vi "Open.vi"(8 "error in":errorcluster, 9 "parameters":variant, 10 "file path":path, 11 "CEF_Hierachy Repository in":refnum<class "CEF_HierarchyRepo.lvclass">) -> (0 "error out":errorcluster, 2 "invalid?":bool, 3 "CEF_Hierachy repository out":refnum<class "CEF_HierarchyRepo.lvclass">)   [LabVIEW 2023, in "CEF.lvlib" / "CEF_HierarchyRepo.lvclass"]
doc: "Loads the saved information of the repo. It could load multiple files at the same time. An option to add file versioning could be included in the files, and the code to manage changes would be in this VI.Copyright 2017 National Instruments Corporation\n\nLicensed under the Apache License, Version 2.0 (the \"License\"); you may not use this file except in compliance with the License. You may obtain a copy of the License at http://www.apache.org/licenses/LICENSE-2.0\nUnless required by applicable law or agreed to in writing, software distributed under the License is distributed on an \"AS IS\" BASIS, WITHOUT WARRANTIES OR CONDITIONS OF ANY KIND, either express or implied. See the License for the specific language governing permissions and limitations under the License."
uses:
  CEF_HierarchyRepo.lvclass
  CEF_HierarchyRepo.lvclass/CEF_HierarchyRepo.ctl
  CEF.lvlib
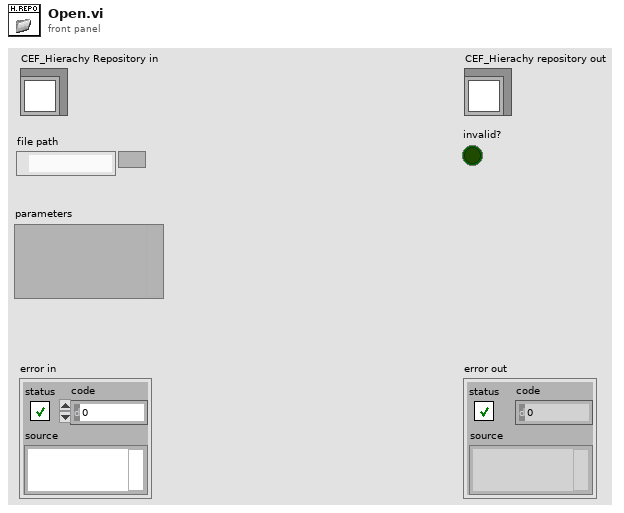
[diagram p1: front panel]
types:
  T1 = typedef "CEF.lvlib/base file format.ctl" = cluster{"version":string, "data":string}
  T2 = typedef "CEF.lvlib/flat hierarchy.ctl" = cluster{"hierarchy structure":T3, "instance data":T5[]}
  T3 = typedef "CEF.lvlib/CEF_HierarchyRepo.lvclass/full hierarchy.ctl" = cluster{"root":string, "hierarchy":T4[]}
  T4 = typedef "CEF.lvlib/hierarchy element.ctl" = cluster{"current node":string, "children":string[]}
  T5 = typedef "CEF.lvlib/instance data.ctl" = cluster{"ID":string, "Alias":string, "class":string, "version":string, "data":string}
  T6 = typedef "CEF.lvlib/CEF_HierarchyRepo.lvclass/memory hierarchy.ctl" = cluster{"hierarchy structure":T3, "instance data":refnum<class "CEF_serializable configuration.lvclass">[]}
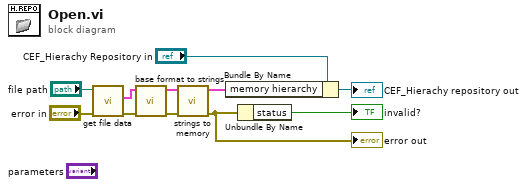
[diagram p0: block diagram]
diagram:
  n1 = call "get file data.vi"("error in"="error in", "Path"="file path") -> ("error out"=w6:errorcluster, "format"=w7:T1)  [unwired: 8 in]
  n2 = call "base format to strings.vi"("error in"=w6, "format"=w7) -> ("error out"=w5:errorcluster, "data"=w4:T2)  [unwired: 8 in]
  n3 = call "strings to memory.vi"("error in"=w5, "1.0.0"=w4) -> ("error out"=w2:errorcluster, "memory hierarchy"=w3:T6)  [unwired: 8 in]
  "error out" <- w2
  n4 = Bundle By Name(cluster="CEF_Hierachy Repository in", "memory hierarchy"=w3) -> (→"CEF_Hierachy repository out":refnum<class "CEF_HierarchyRepo.lvclass">)
  n5 = Unbundle By Name(w2) -> ("status"=→"invalid?":bool)
